vi "Stage 3.6 Placing init and close into subVIs.vi"() -> ()   [LabVIEW 2020]
panel:
  out "Process Error":errorcluster
  out "error out":errorcluster
  out "error out Hardware":errorcluster
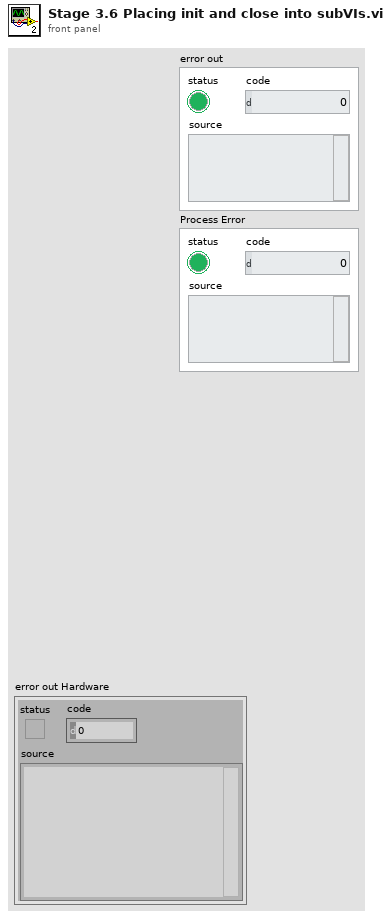
[diagram p1: front panel]
types:
  T1 = typedef "HRM-Stage3-init_cluster.ctl" = cluster{"User events":T2}
  T2 = typedef "HRM-Stage3-User_events.ctl" = cluster{"Signal to remove":refnum<user-event>, "Sample size":refnum<user-event>, "Filtered wf":refnum<user-event>, "Unfiltered wf":refnum<user-event>, "Raw wf":refnum<user-event>, "Pulse":refnum<user-event>, "Stop":refnum<user-event>}
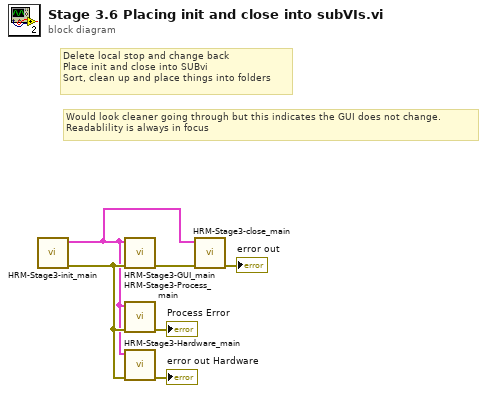
[diagram p0: block diagram]
diagram:
  # "Would look cleaner going through but this indicates the GUI does not change.\nReadablility is always in focus"
  # "Delete local stop and change back\nPlace init and close into SUBvi\nSort, clean up and place things into folders"
  n1 = call "HRM-Stage3-init_main.vi"() -> ("error out"=w3:errorcluster, "Init cluster"=w1:T1)  [unwired: 10 in]
  n2 = call "HRM-Stage3-GUI_main.vi"("error in (no error)"=w3, "Init cluster"=w1) -> ("error out"=w2:errorcluster)  [unwired: 9 in]
  n3 = call "HRM-Stage3-Process_main.vi"("error in (no error)"=w3, "Init cluster"=w1) -> ("error out"=→"Process Error":errorcluster)  [unwired: 9 in]
  n4 = call "HRM-Stage3-Hardware_main.vi"("error in (no error)"=w3, "Init cluster"=w1) -> ("error out"=→"error out Hardware":errorcluster)  [unwired: 9 in]
  n5 = call "HRM-Stage3-close_main.vi"("error in (no error)"=w2, "Init cluster"=w1) -> ("error out"=→"error out":errorcluster)  [unwired: 9 in]
